vi "ExtractIcon.vi"(4 "error in (no error)":errorcluster, 6 "IconIndex (0)":i32, 7 "Path to Icon file (*.exe, *.dll, *.ico)":path) -> (0 "error out":errorcluster, 3 "hIcon":i32)   [LabVIEW 2011]
uses:
  SHELL32.DLL
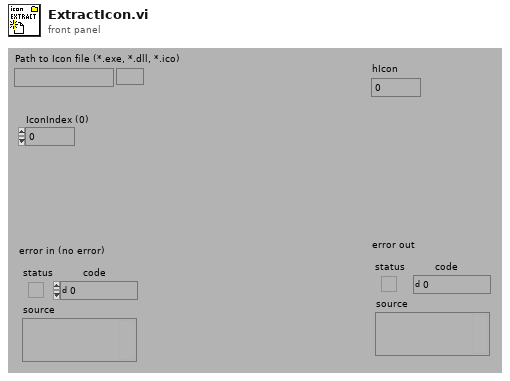
[diagram p1: front panel]
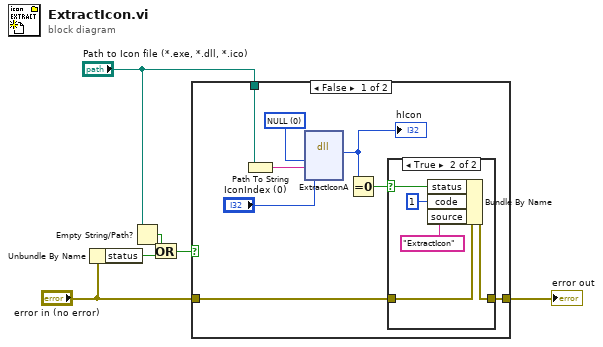
[diagram p0: block diagram]
diagram:
  n1 = Unbundle By Name("error in (no error)") -> ("status"=w4:bool)
  n2 = Empty String/Path?(string/path="Path to Icon file (*.exe, *.dll, *.ico)") -> (empty?=w5:bool)
  n3 = Or(x=w5, y=w4) -> (x .or. y?=w1:bool)
  n4 = case shown="False" w1 {
    tunnel: "Path to Icon file (*.exe, *.dll, *.ico)" -> [w14 _]
    tunnel: [w9 w21] -> w6
    tunnel: "error in (no error)" -> [w8 w21]
    frame False {
      w12 = 0 items=["NULL"]
      n5 = Path To String(path=w14) -> (string=w13:string)
      n6 = dll-call lib="SHELL32.DLL" fn="ExtractIconA"("hInst"=w12, "lpszIconFileName"=w13, "nIconIndex"="IconIndex (0)") -> (w11:i32)  [unwired: 6 in, 2 out]
      "hIcon" <- w11
      n7 = Equal To 0?(x=w11) -> (x = 0?=w10:bool)
      n8 = case shown="True" w10 {
        selector: w10 -> [_ w19]
        tunnel: w8 -> [w15 w20]
        tunnel: [w15 w16] -> w9
        frame False {
        }
        frame True {
          n9 = Bundle By Name(cluster=w20, "status"=w19, "code"=1, "source"="ExtractIcon") -> (w16:errorcluster)
        }
      }
    }
    frame True {
    }
  }
  "error out" <- w6
